vi "Configure INTERLOCK Mode.vi"(8 "error in (no error)":errorcluster, 10 "Interlock mode":string(combo)="OPEN", 11 "BoardHandle":T1) -> (0 "error out":errorcluster, 3 "BoardHandle out":T1)   [LabVIEW 2009, in "CAEN PSM.lvlib"]
doc: "This function allows to select Interlock logic."
uses:
  <instrlib>/CAEN PSM/CAEN PSM.lvlib
  <instrlib>/CAEN PSM/Private/BoardHandle.ctl
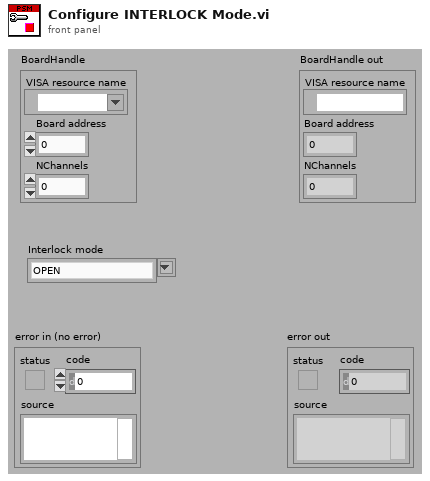
[diagram p1: front panel]
types:
  T1 = typedef "CAEN PSM.lvlib/BoardHandle.ctl" = cluster{"VISA resource name":refnum<visa-resource-name>, "Board address":u8, "NChannels":u8}
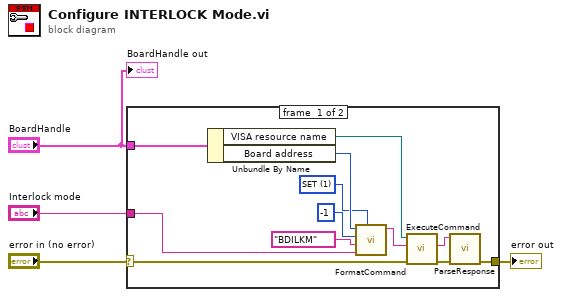
[diagram p0: block diagram]
diagram:
  n1 = case shown="No Error" "error in (no error)" {
    selector: "error in (no error)" -> [w8 w17]
    tunnel: [w11 w17] -> w3
    tunnel: "BoardHandle" -> [w9 _]
    tunnel: "Interlock mode" -> [w6 _]
    frame #0 {
      w15 = u8 1 items=["MON", "SET"] ("CMD")
      n2 = Unbundle By Name(w9) -> ("VISA resource name"=w14:refnum<visa-resource-name>, "Board address"=w16:u8)
      n3 = call <instrlib>:"FormatCommand.vi"("CMD (MON)"=w15, "VAL"=w6, "PAR"="BDILKM", "CH"=i8 -1, "BD (0)"=w16) -> ("cmd"=w13:string)  [unwired: 6 in]
      n4 = call <instrlib>:"ExecuteCommand.vi"("error in (no error)"=w8, "Command"=w13, "VISA resource name"=w14) -> ("error out"=w12:errorcluster, "Response"=w10:string)  [unwired: 6 in, 1 out]
      n5 = call <instrlib>:"ParseResponse.vi"("error in (no error)"=w12, "Response"=w10) -> ("error out"=w11:errorcluster)  [unwired: 6 in, 3 out]
    }
    frame #1 {
    }
  }
  "error out" <- w3
  "BoardHandle out" <- "BoardHandle"
